vi "Launch Log Man.vi"(8 "error in (no error)":errorcluster, 10 "Log Config Path":path, 11 "Caller Actor in":refnum<class "Actor.lvclass">) -> (0 "error out":errorcluster, 3 "Caller Actor out":refnum<class "Actor.lvclass">)   [LabVIEW 2020, in "Logging.lvlib"]
uses:
  Logging.lvlib
  <vilib>/ActorFramework/Actor/Actor.lvclass
  Logger Mananger/Logger Mananger.lvclass
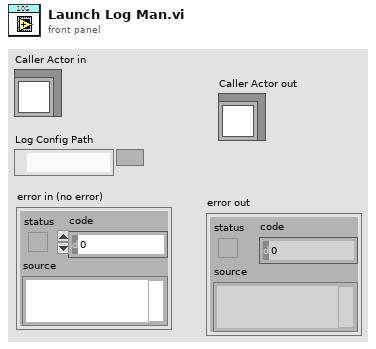
[diagram p1: front panel]
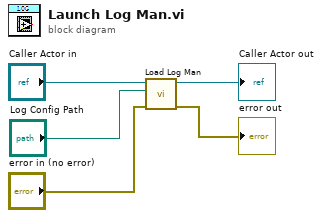
[diagram p0: block diagram]
diagram:
  n1 = call "Load Log Man.vi"("error in (no error)"="error in (no error)", "Log Config Path"="Log Config Path", "Caller Actor in"="Caller Actor in") -> ("error out"=→"error out":errorcluster, "Caller Actor out"=→"Caller Actor out":refnum<class "Actor.lvclass">)  [unwired: 7 in]
